vi "Host Main.vi"() -> ()   [LabVIEW 2017]
panel:
  in  "Stop Button":bool
  out "Waveform Chart":i32(graph)
  out "error out":errorcluster
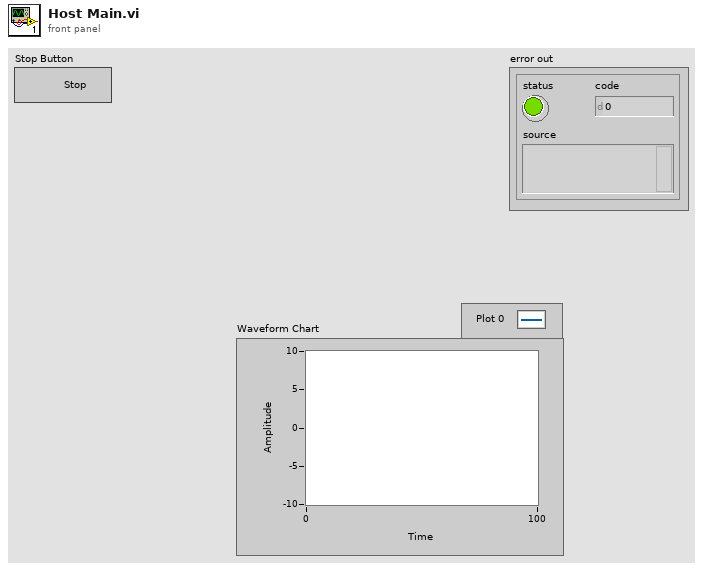
[diagram p1: front panel]
types:
  T1 = enum16{"open", "replace", "create", "open or create", "replace or create", "replace or create with confirmation"}
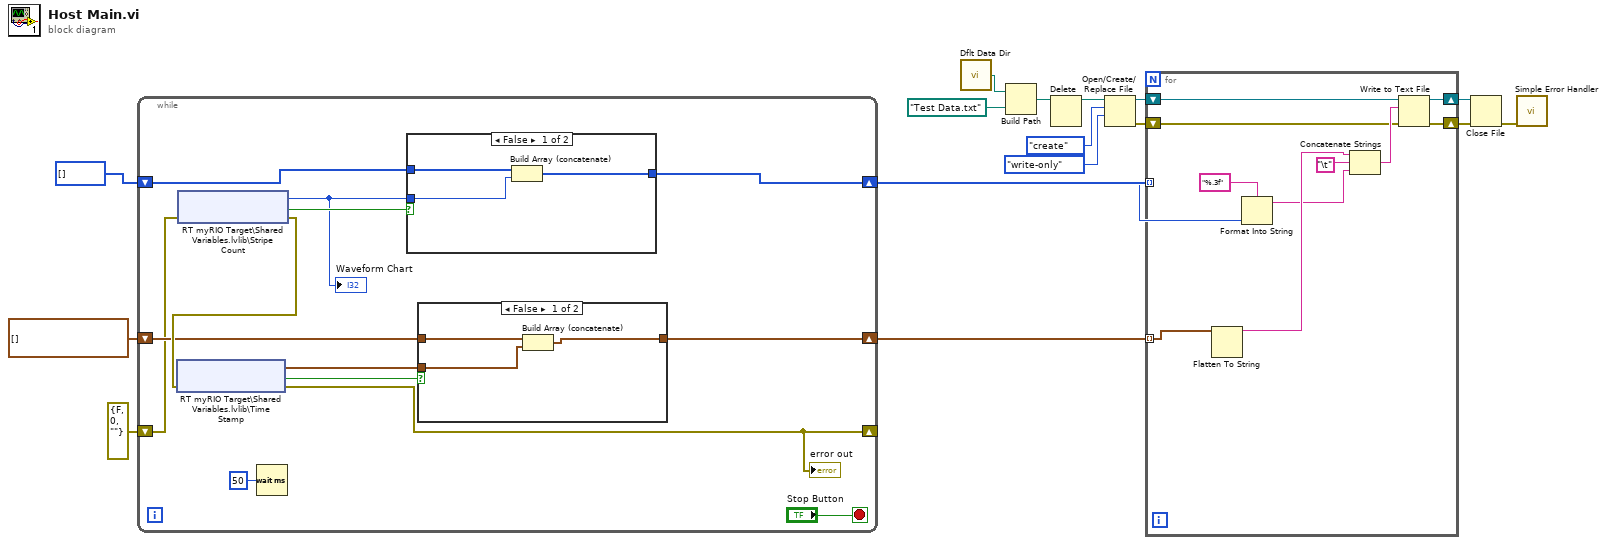
[diagram p0: block diagram]
diagram:
  n1 = while {
    shift-right: [w25] -> w2
    shift-left: i32[] [] -> [w27]
    shift-right: [w23] -> w1
    shift-left: timestamp[] [] -> [w22]
    shift-right: [w19] -> _
    shift-left: errorcluster {"status"=FALSE, "code"=0, "source"=""} ("error IO") -> [w20]
    stop <- "Stop Button" stop-if-true
    n2 = shared-variable "RT myRIO Target\\Shared Variables.lvlib\\Stripe Count"(error in=w20) -> (w18:i32, error out=w28:errorcluster, w26:bool)  [unwired: 1 in]
    "Waveform Chart" <- w18
    n3 = shared-variable "RT myRIO Target\\Shared Variables.lvlib\\Time Stamp"(error in=w28) -> (w24:timestamp, error out=w19:errorcluster, w21:bool)  [unwired: 1 in]
    "error out" <- w19
    n4 = Wait (ms)(milliseconds to wait=u32 50) -> ()  [unwired: 1 out]
    n5 = case shown="False" w26 {
      tunnel: w27 -> [w36 w37]
      tunnel: [w34 w37] -> w25
      tunnel: w18 -> [w35 _]
      frame False {
        n6 = Build Array (concatenate)(w36, w35) -> (w34:i32[])
      }
      frame True {
      }
    }
    n7 = case shown="False" w21 {
      tunnel: [w31 w33] -> w23
      tunnel: w24 -> [w32 _]
      tunnel: w22 -> [w30 w33]
      frame False {
        n8 = Build Array (concatenate)(w30, w32) -> (w31:timestamp[])
      }
      frame True {
      }
    }
  }
  n9 = call <vilib>:"Dflt Data Dir.vi"() -> ("App:Default Data Directory"=w4:path)
  n10 = Build Path(base path=w4, name or relative path=path "Test Data.txt" ("default name")) -> (appended path=w6:path)
  n11 = Delete(path (use dialog)=w6) -> (deleted path=w3:path)  [unwired: 4 in, 2 out]
  n12 = Open/Create/Replace File(file path (use dialog)=w3, operation (0:open)=T1."create", access (0:read/write)=enum16{"read/write", "read-only", "write-only"}."write-only") -> (refnum out=w10:refnum<file>, error out=w9:errorcluster)  [unwired: 1 in, 3 out]
  n13 = for {
    shift-right: [w47] -> w13
    shift-left: w10 -> [w45]
    shift-right: [w44] -> w12
    shift-left: w9 -> [w41]
    tunnel: w2 -> [w38] mode=indexing
    tunnel: w1 -> [w43] mode=indexing
    n14 = Flatten To String(anything=w43) -> (data string=w42:string)  [unwired: 3 in, 2 out]
    n15 = Format Into String(format string="%.3f", w38) -> (resulting string=w39:string)  [unwired: 2 in, 1 out]
    n16 = Concatenate Strings(w42, "\t" ("Tab"), w39) -> (w46:string)
    n17 = Write to Text File(file (use dialog)=w45, text=w46, error in=w41) -> (refnum out=w47:refnum<file>, error out=w44:errorcluster)  [unwired: 1 in, 1 out]
  }
  n18 = Close File(refnum=w13, error in=w12) -> (error out=w11:errorcluster)  [unwired: 1 out]
  n19 = call <vilib>:"Simple Error Handler.vi"("error in (no error)"=w11) -> ()  [unwired: 1 in, 8 out]
